vi "ArmGetPresets.vi"(10 "Game Piece":T2, 11 "Position":T1=enum."Middle") -> (1 "z":dbl, 3 "x":dbl)   [LabVIEW 2020]
uses:
  ArmGamePiecePreset.ctl
  ArmPositionPreset.ctl
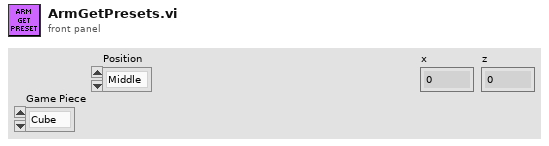
[diagram p1: front panel]
types:
  T1 = typedef "ArmPositionPreset.ctl" = enum16{"Upper", "Lower", "Middle", "Home", "Shelf", "Floor", "HalfFloor", "HalfHome"}
  T2 = typedef "ArmGamePiecePreset.ctl" = enum16{"Cube", "Cone"}
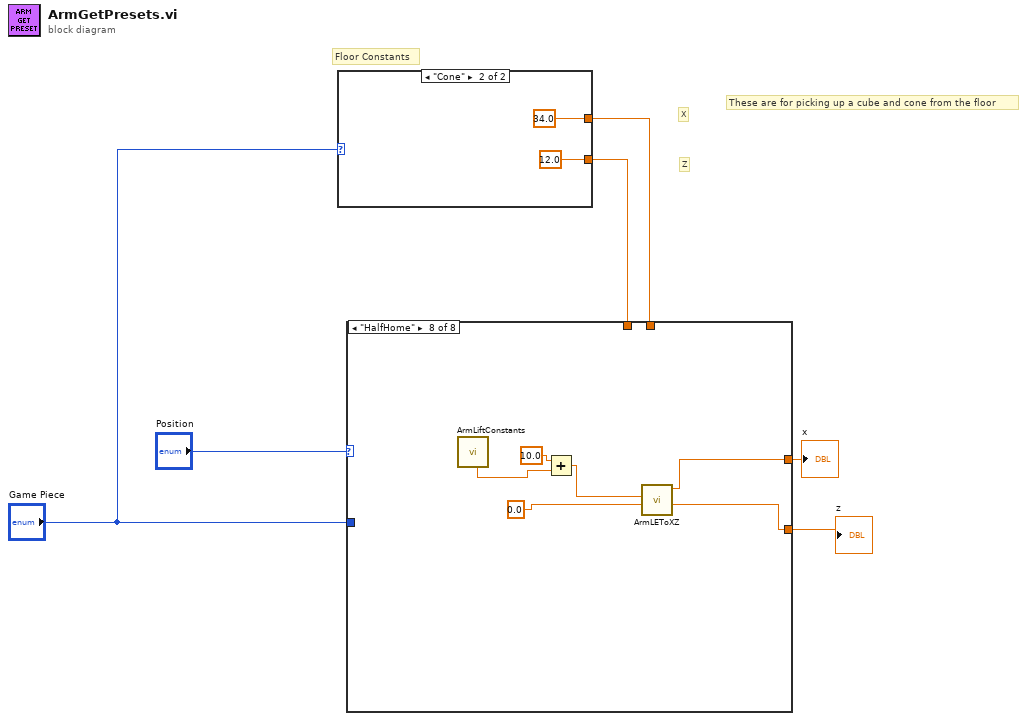
[diagram p0: block diagram]
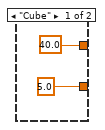
[diagram p2: hidden frame]
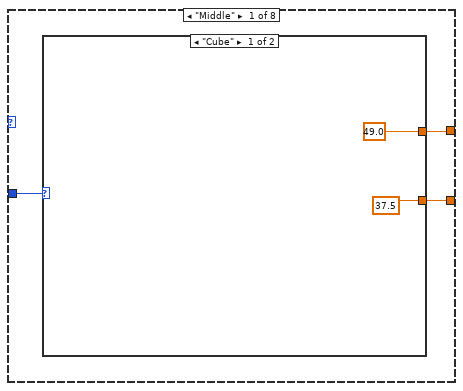
[diagram p3: hidden frame]
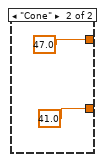
[diagram p4: hidden frame]
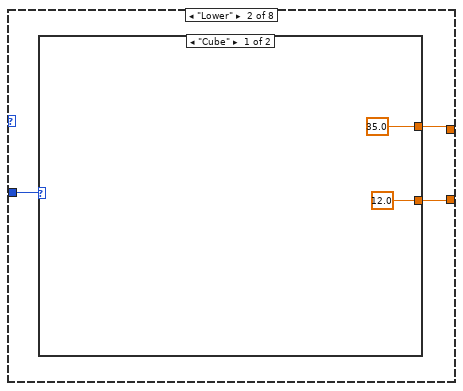
[diagram p5: hidden frame]
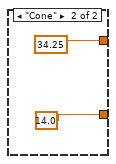
[diagram p6: hidden frame]
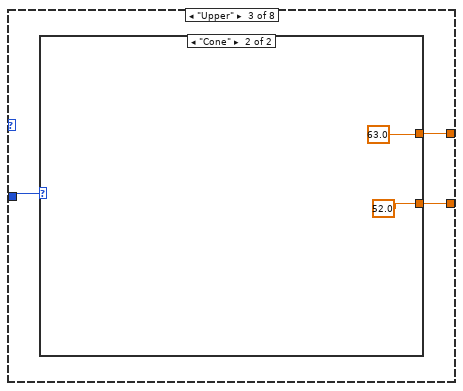
[diagram p7: hidden frame]
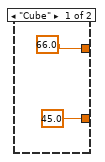
[diagram p8: hidden frame]
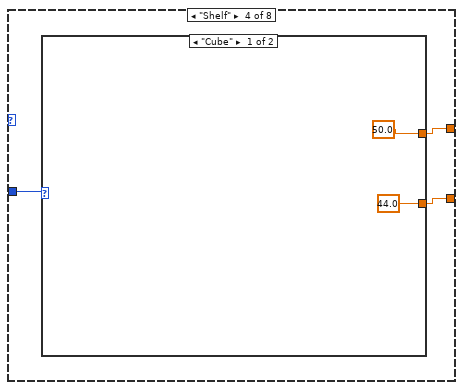
[diagram p9: hidden frame]
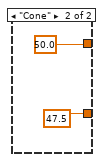
[diagram p10: hidden frame]
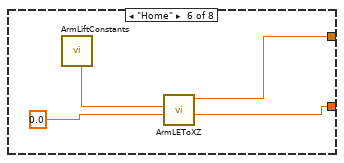
[diagram p12: hidden frame]
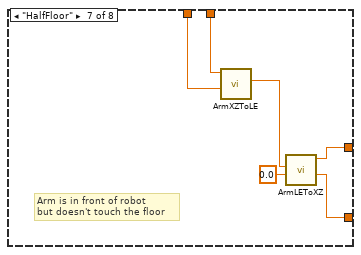
[diagram p13: hidden frame]
diagram:
  # "These are for picking up a cube and cone from the floor"
  # "Z"
  # "X"
  # "Floor Constants"
  n1 = case shown="\"Cone\"" "Game Piece" {
    tunnel: [40.0 34.0] -> w3
    tunnel: [5.0 12.0] -> w2
    frame "Cube" {
    }
    frame "Cone" {
    }
  }
  n2 = case shown="\"HalfHome\"" "Position" {
    tunnel: [w12 w20 w27 w33 w40 w42 w48 w55] -> w6
    tunnel: [w11 w19 w26 w32 w39 w41 w47 w54] -> w5
    tunnel: "Game Piece" -> [w13 w18 w25 w34 _ _ _ _]
    tunnel: w3 -> [_ _ _ _ w40 _ w46 _]
    tunnel: w2 -> [_ _ _ _ w39 _ w45 _]
    frame "Middle" {
      n3 = case shown="\"Cube\"" w13 {
        tunnel: [49.0 47.0] -> w12
        tunnel: [37.5 41.0] -> w11
        frame "Cube" {
        }
        frame "Cone" {
        }
      }
    }
    frame "Lower" {
      n4 = case shown="\"Cube\"" w18 {
        tunnel: [35.0 34.25] -> w20
        tunnel: [12.0 14.0] -> w19
        frame "Cube" {
        }
        frame "Cone" {
        }
      }
    }
    frame "Upper" {
      n5 = case shown="\"Cone\"" w25 {
        tunnel: [66.0 63.0] -> w27
        tunnel: [45.0 52.0] -> w26
        frame "Cube" {
        }
        frame "Cone" {
        }
      }
    }
    frame "Shelf" {
      n6 = case shown="\"Cube\"" w34 {
        tunnel: [50.0 50.0] -> w33
        tunnel: [44.0 47.5] -> w32
        frame "Cube" {
        }
        frame "Cone" {
        }
      }
    }
    frame "Floor" {
    }
    frame "Home" {
      n7 = call "ArmLiftConstants.vi"() -> ("Default Angle"=w44:dbl)  [unwired: 8 in, 3 out]
      n8 = call "ArmLEToXZ.vi"("Extend"=0.0, "Lift"=w44) -> ("z"=w41:dbl, "x"=w42:dbl)  [unwired: 8 in]
    }
    frame "HalfFloor" {
      # "Arm is in front of robot\nbut doesn't touch the floor"
      n9 = call "ArmXZToLE.vi"("Z"=w45, "X"=w46) -> ("Lift"=w49:dbl)  [unwired: 8 in, 1 out]
      n10 = call "ArmLEToXZ.vi"("Extend"=0.0, "Lift"=w49) -> ("z"=w47:dbl, "x"=w48:dbl)  [unwired: 8 in]
    }
    frame "HalfHome" {
      n11 = call "ArmLiftConstants.vi"() -> ("Default Angle"=w53:dbl)  [unwired: 8 in, 3 out]
      n12 = Add(x=10.0, y=w53) -> (x+y=w51:dbl)
      n13 = call "ArmLEToXZ.vi"("Extend"=0.0, "Lift"=w51) -> ("z"=w54:dbl, "x"=w55:dbl)  [unwired: 8 in]
    }
  }
  "x" <- w6
  "z" <- w5
